vi "Subscribe to Broadcast.vi"(8 "error in (no error)":errorcluster, 11 "API-Reference in":refnum<data-value>) -> (0 "error out":errorcluster, 3 "API-Reference out":refnum<data-value>)   [LabVIEW 2018]
uses:
  Actor.lvclass
  Stopped.ctl
  Stop.ctl
  Message-Enqueue Refs.ctl
  API-Data.ctl
  Did Initialize.ctl
  Launch.ctl
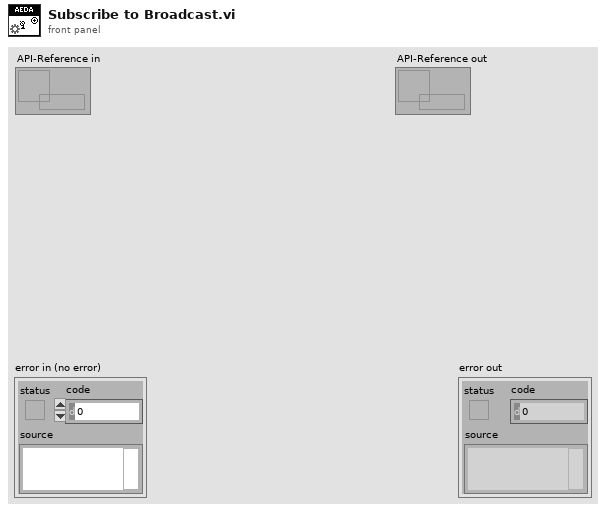
[diagram p1: front panel]
types:
  T1 = typedef "Actor.lvclass/API-Data.ctl" = cluster{"Launch":refnum<notifier>, "Did Stop Enqueuer":refnum<user-event>, "Message Enqueuers":T2, "Stopped Reg":refnum<event-registration>}
  T2 = typedef "Actor.lvclass/Message-Enqueue Refs.ctl" = cluster{"Stop":refnum<user-event>, "Launch":refnum<user-event>, "Did Initialize":refnum<user-event>}
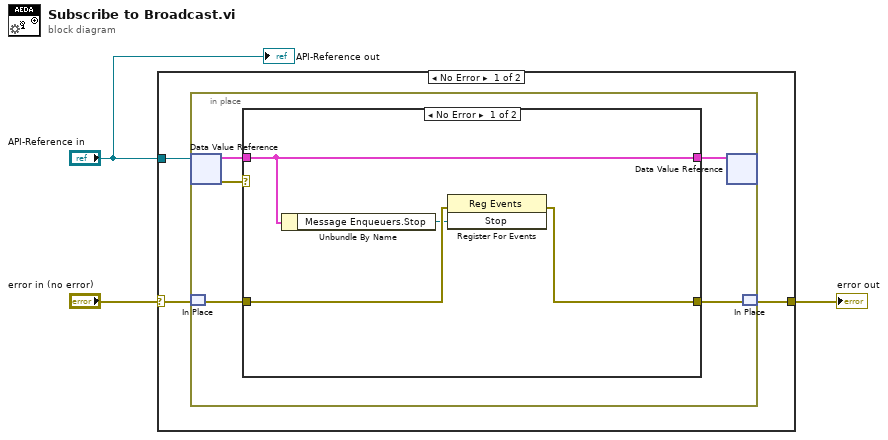
[diagram p0: block diagram]
diagram:
  n1 = case shown="No Error" "error in (no error)" {
    selector: "error in (no error)" -> [w6 w18]
    tunnel: [w5 w18] -> w2
    tunnel: "API-Reference in" -> [w4 _]
    frame No Error {
      n2 = in-place {
        n3 = in-place-dvr #1(w4) -> (w10:T1, w11:errorcluster)
        n4 = in-place-match #2(w6) -> (w8:errorcluster)
        n5 = case shown="No Error" w11 {
          selector: w11 -> [_ w17]
          tunnel: w10 -> [w12 w16]
          tunnel: [w12 w16] -> w9
          tunnel: w8 -> [w15 _]
          tunnel: [w14 w17] -> w7
          frame No Error {
            n6 = Unbundle By Name(w12) -> ("Message Enqueuers.Stop"=w13:refnum<user-event>)
            n7 = register-events(error in=w15, w13) -> (error out=w14:errorcluster)  [unwired: 1 in, 1 out]
          }
          frame Error {
          }
        }
        n8 = in-place-dvr #1(w9) -> ()  [unwired: 2 out]
        n9 = in-place-match #2(w7) -> (w5:errorcluster)
      }
    }
    frame Error {
    }
  }
  "error out" <- w2
  "API-Reference out" <- "API-Reference in"
